vi "AFM_DLog.LogSettingsToDataBase.vi"(4 "Interpolation":dbl format="%#_13g", 6 "Writing Setpoint":dbl format="%#_13g", 8 "error in (no error)":errorcluster, 9 "Amplifier":dbl format="%#_13g", 10 "Move Setpoint":dbl format="%#_13g", 11 "Instrument.AFM_DLog in":refnum<class "Instrument.AFM_DLog.lvclass">) -> (0 "error out":errorcluster, 3 "Instrument.AFM_DLog out":refnum<class "Instrument.AFM_DLog.lvclass">)   [LabVIEW 2019, in "Instrument.AFM_DLog.lvclass"]
uses:
  Instrument.AFM_DLog.lvclass
  C:/Program Files (x86)/National Instruments/LabVIEW 2019/user.lib/LevyLab/Instrument Framework/Instrument/Instrument.lvclass
  <userlib>/LevyLab/Instrument Framework/Instrument/Instrument.lvclass
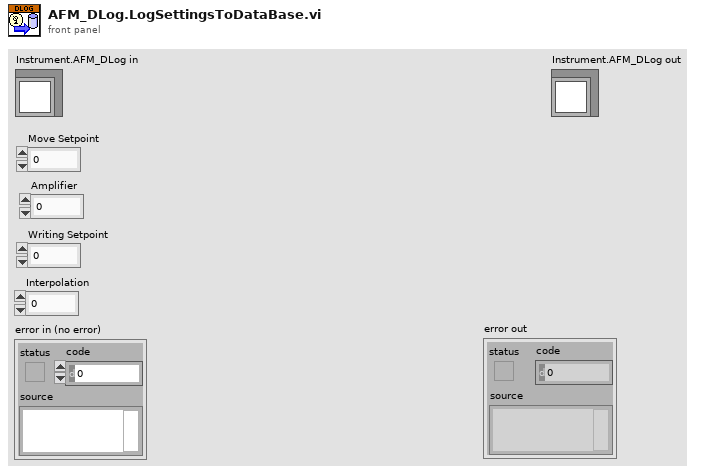
[diagram p1: front panel]
types:
  T1 = cluster{"Move Setpoint":dbl, "Amplifier":dbl, "Writing Setpoint":dbl, "Interpolation":dbl}
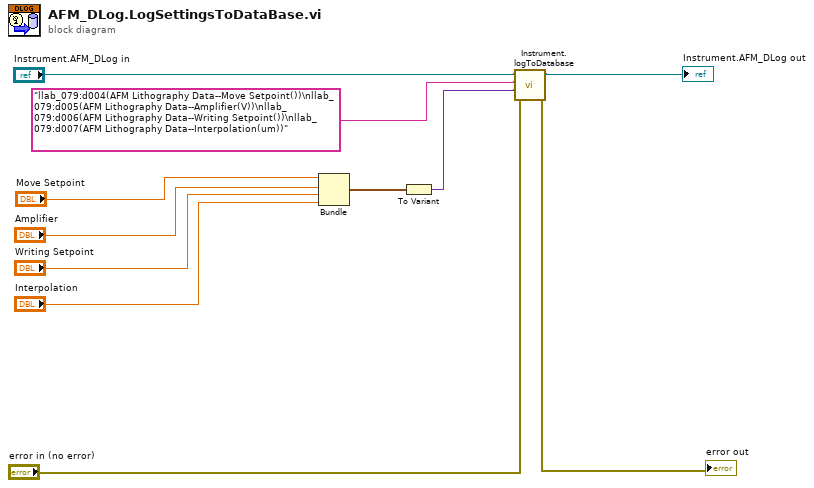
[diagram p0: block diagram]
diagram:
  n1 = Bundle("Move Setpoint"="Move Setpoint", "Amplifier"="Amplifier", "Writing Setpoint"="Writing Setpoint", "Interpolation"="Interpolation") -> (w6:T1)  [unwired: 1 in]
  n2 = To Variant(anything=w6) -> (Variant=w5:variant)
  n3 = call <userlib>:"Instrument.logToDatabase.vi"("error in (no error)"="error in (no error)", "Data"=w5, "Paths"="llab_079:d004(AFM Lithography Data--Move Setpoint())\nllab_079:d005(AFM Lithography Data--Amplifier(V))\nllab_079:d006(AFM Lithography Data--Writing Setpoint())\nllab_079:d007(AFM Lithography Data--Interpolation(um))", "Instrument"="Instrument.AFM_DLog in") -> ("error out"=→"error out":errorcluster, "Instrument out"=→"Instrument.AFM_DLog out":refnum<class "Instrument.AFM_DLog.lvclass">)  [unwired: 6 in]
